vi "UI Andor.vi"(8 "error in":errorcluster) -> (0 "error out":errorcluster)   [LabVIEW 2019, in "Andor.lvlib"]
uses:
  Andor.lvlib
  User Event/Controls/UE Abort Action.ctl
  <vilib>/vision/Image Controls.llb/IMAQ Image.ctl
  <vilib>/Utility/miscctls.llb/LVPointTypeDef.ctl
  <vilib>/Utility/error.llb/Error Cluster From Error Code.vi
  <vilib>/ErrorRing/Error Ring.xnode
  Queues/Queues.lvlib
panel:
  in  "Overlay":bool
  in  "Exposure Time(s)":dbl=0.05 min=0.01 max=5.0
  out "Image":T1(plugin-control)
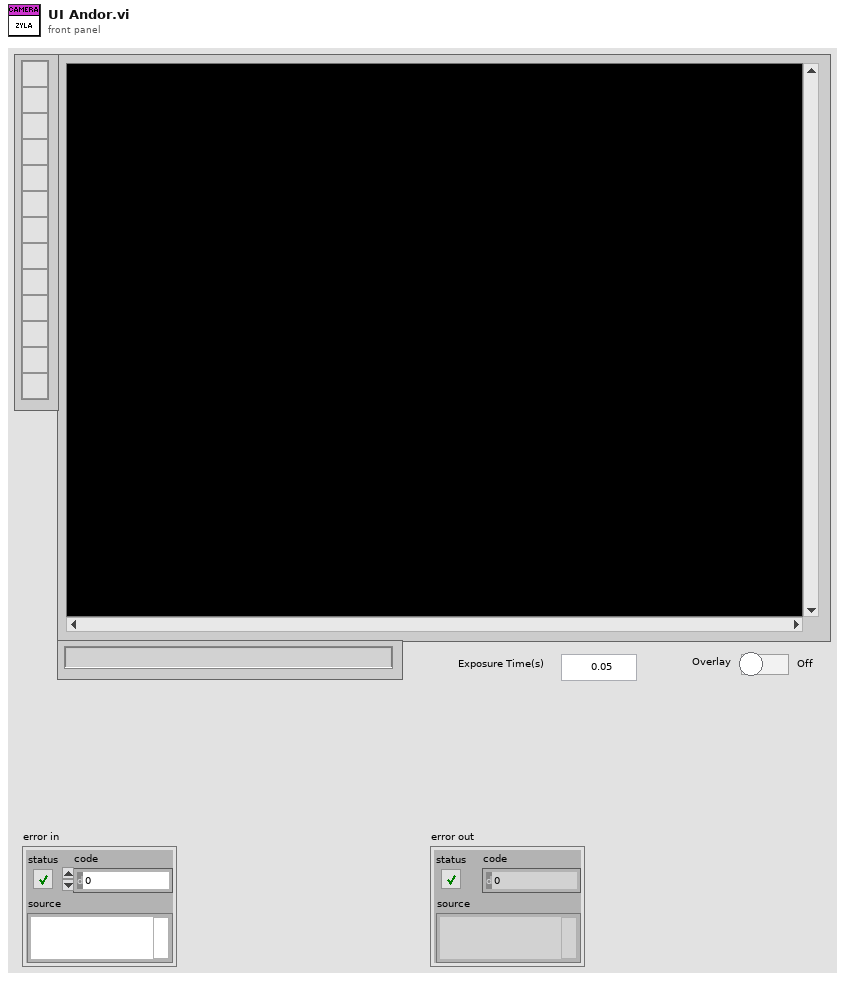
[diagram p1: front panel]
types:
  T1 = typedef "IMAQ Image.ctl" = refnum<image>
  T2 = typedef "IMAQ Point" = cluster{"X":sgl, "Y":sgl}
  T3 = cluster{"Image(U16)":T1, "Initialize Sucess?":bool, "Cursor Points":T2[], "Overlay?":bool}
  T4 = typedef "UE Abort Action.ctl" = enum16{"Create", "Get", "Destroy"}
  T5 = typedef "LVPointTypeDef.ctl" = cluster{"Horizontal":i16, "Vertical":i16}
  T6 = enum16{"Initial", "Start", "Astop", "Snap", "Exposure", "Close"}
  T7 = typedef "Image Type" = u32
  T8 = typedef "Andor.lvlib/SEQ Data.ctl" = cluster{"Initialize Sucess?":bool, "Image Ref":T1, "VI Refnum":refnum<vi>}
  T9 = typedef "Rendezvous RefNum" = refnum<k1>
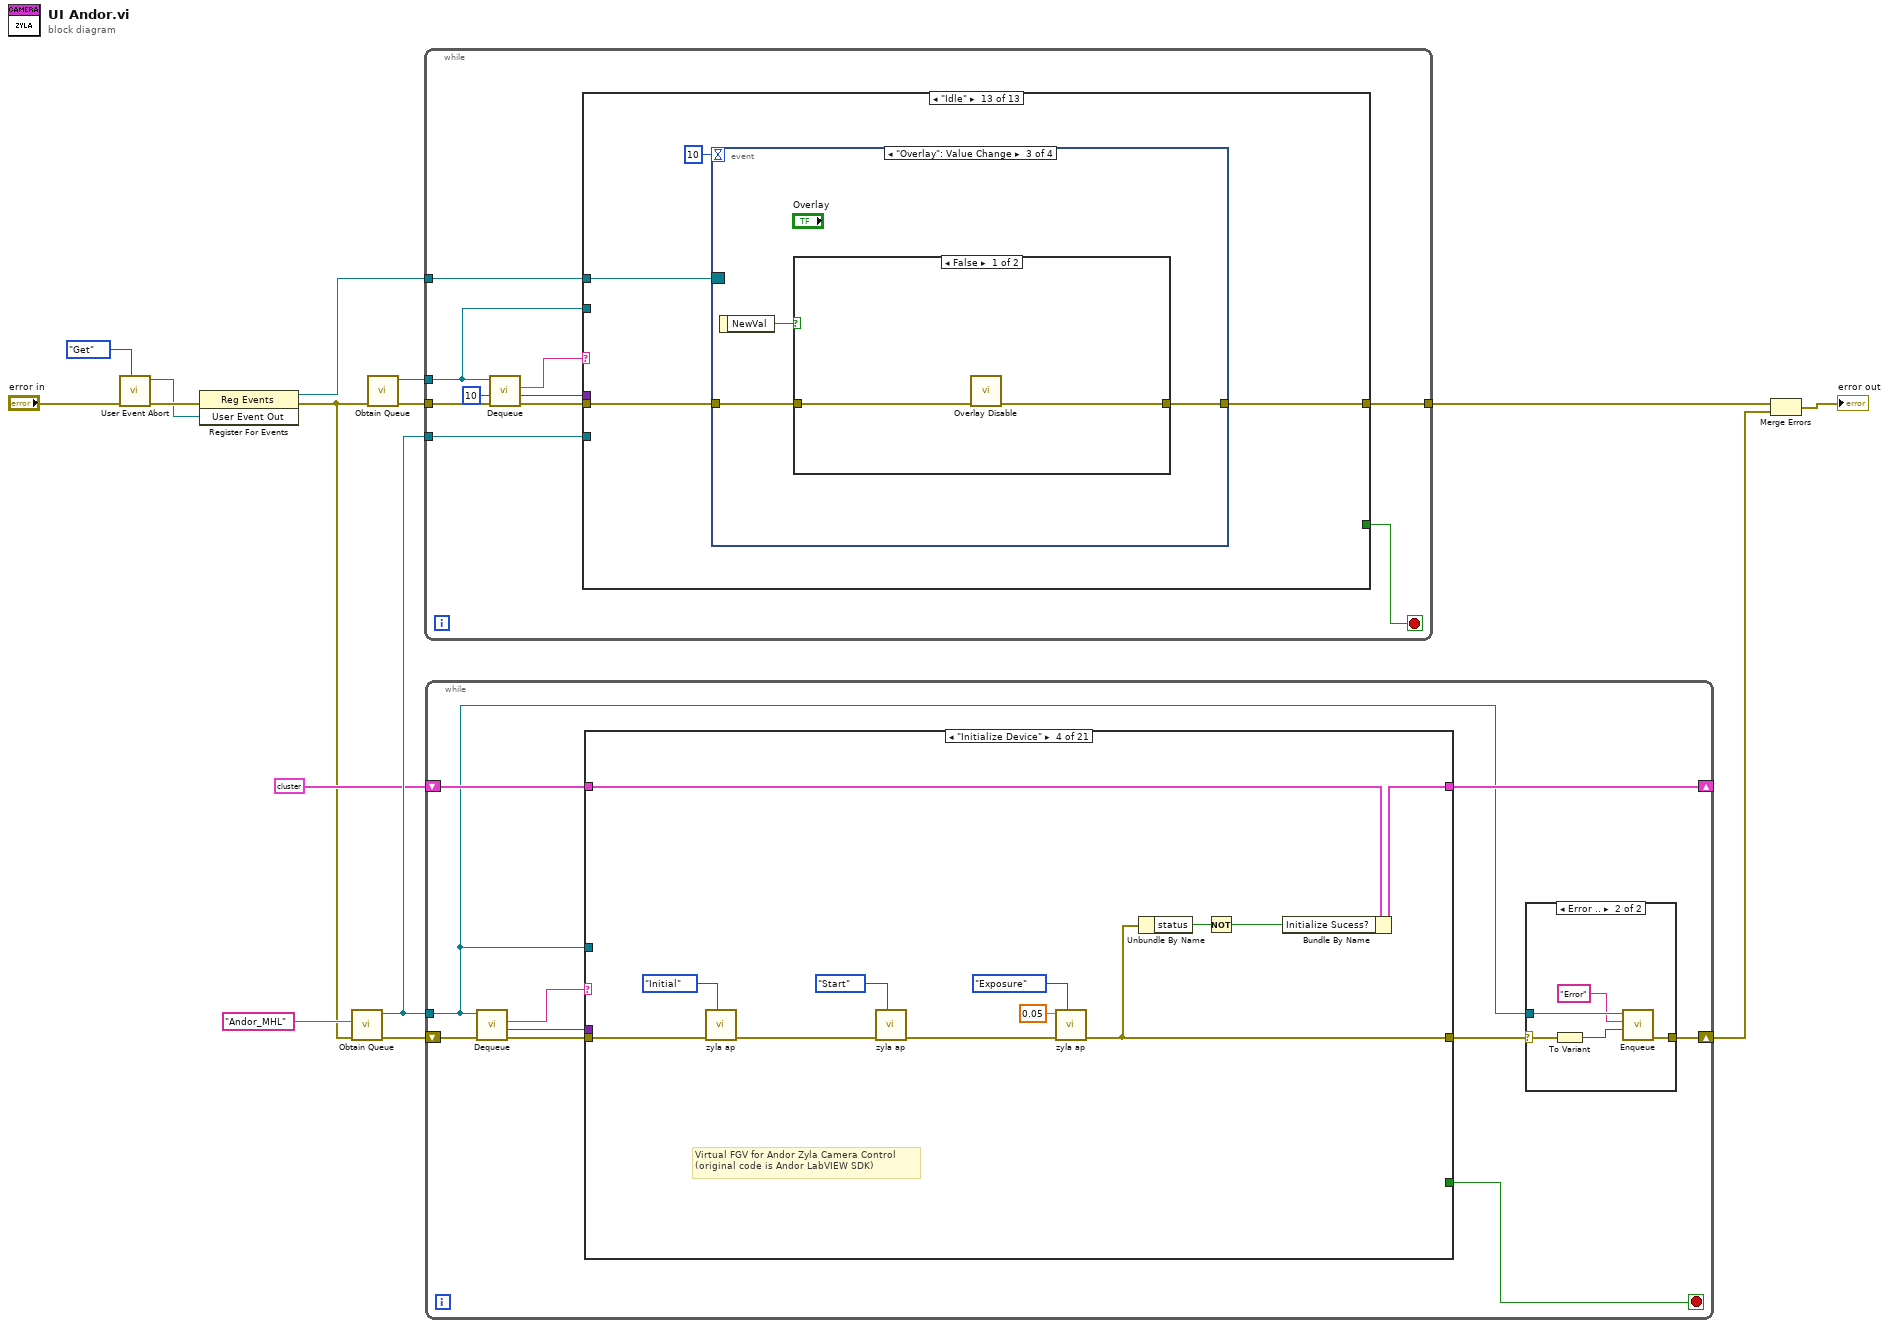
[diagram p0: block diagram]
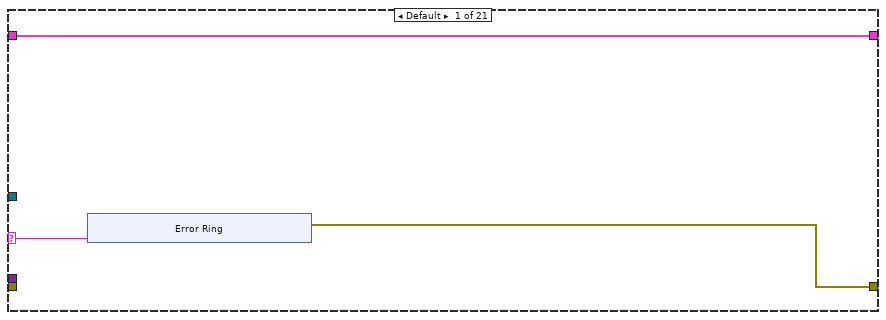
[diagram p2: hidden frame]
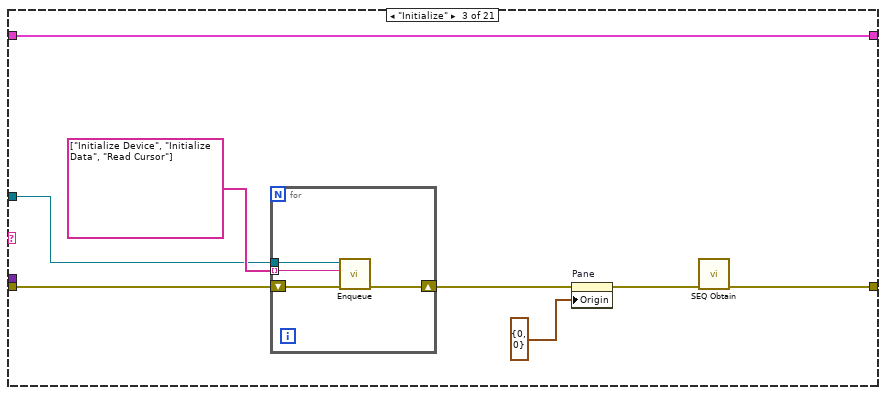
[diagram p4: hidden frame]
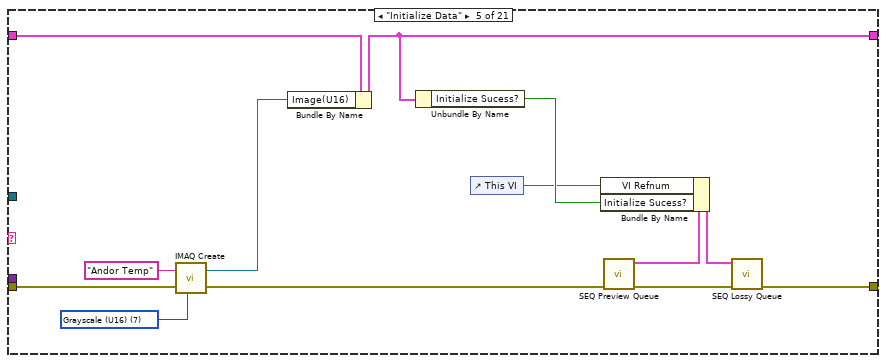
[diagram p5: hidden frame]
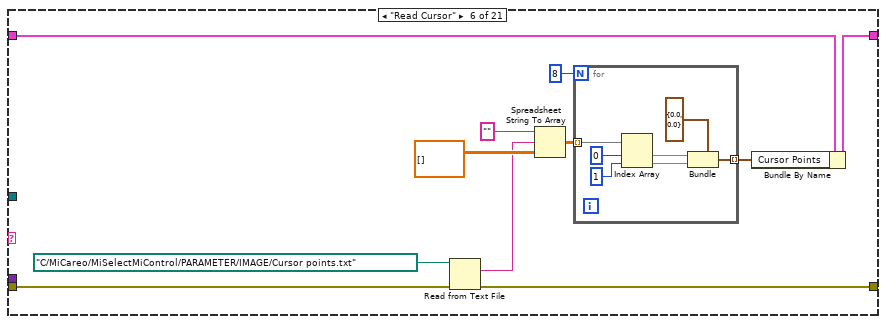
[diagram p6: hidden frame]
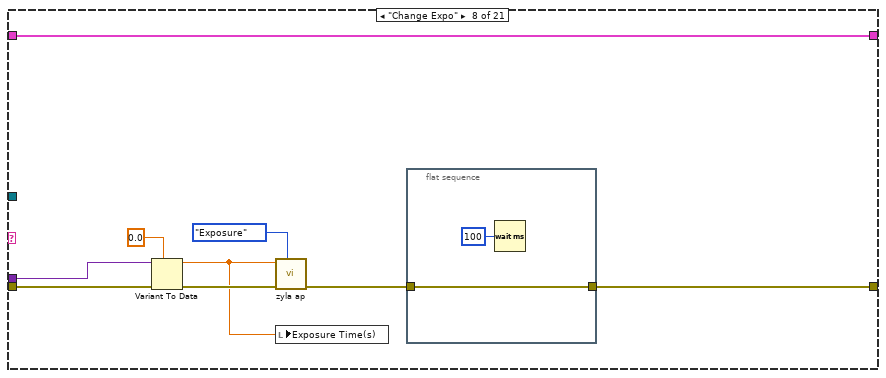
[diagram p8: hidden frame]
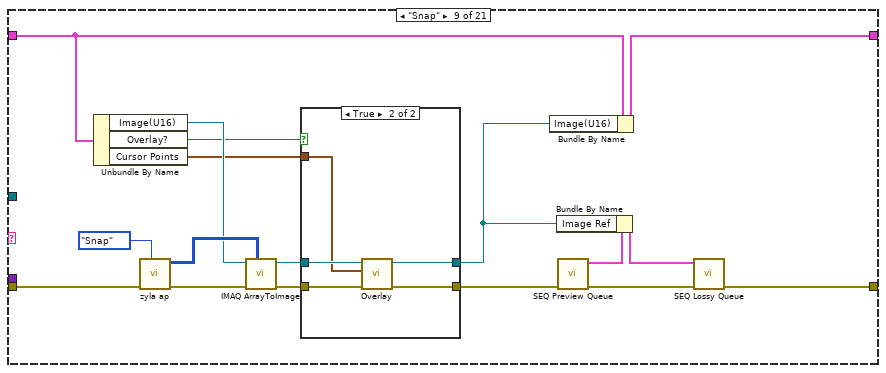
[diagram p9: hidden frame]
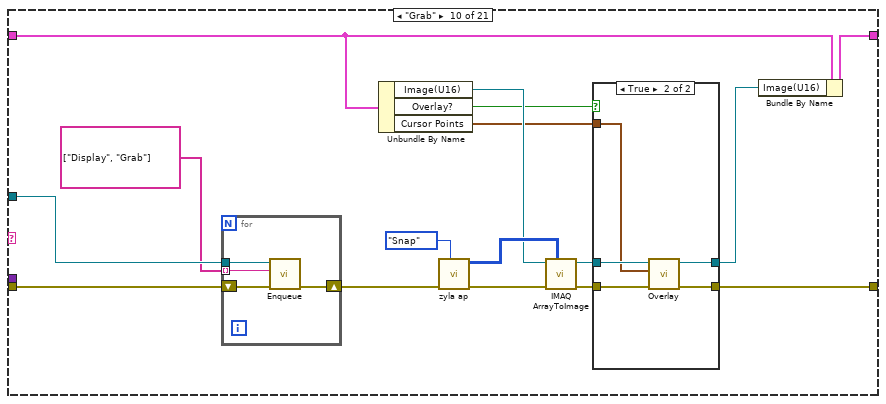
[diagram p11: hidden frame]
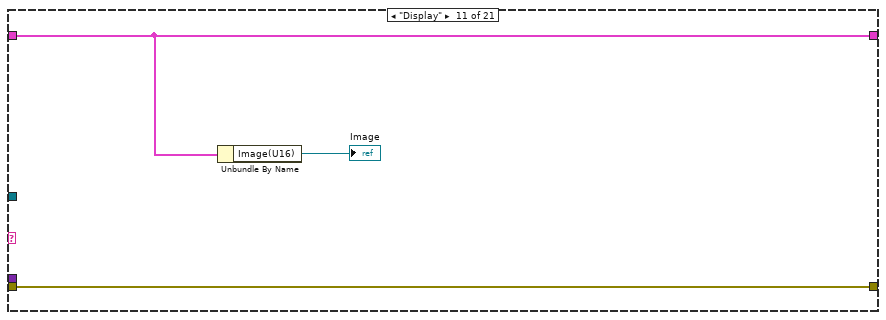
[diagram p13: hidden frame]
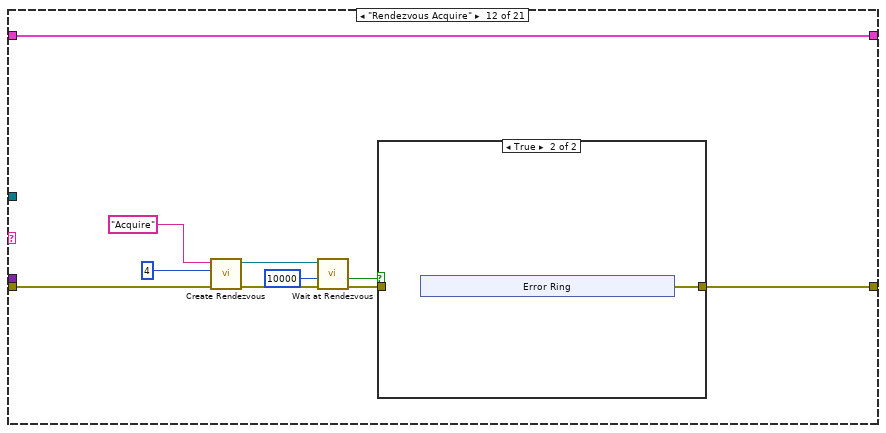
[diagram p14: hidden frame]
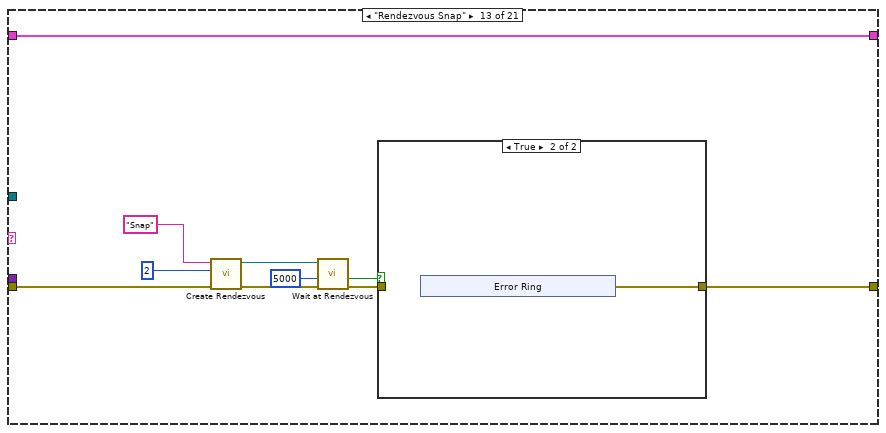
[diagram p16: hidden frame]
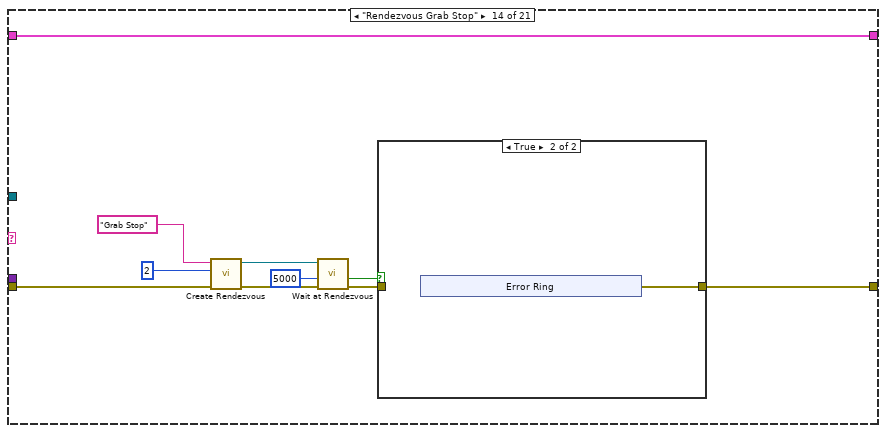
[diagram p18: hidden frame]
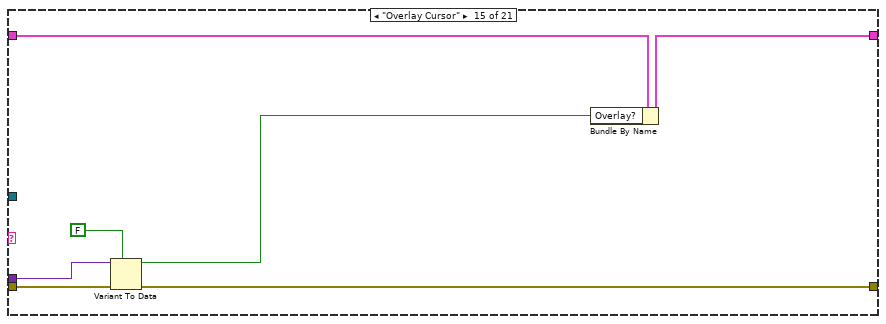
[diagram p20: hidden frame]
diagram:
  n1 = call "User Event Abort.vi"("Action"=UE_Abort_Action."Get", "Error In"="error in") -> ("Error Out"=w13:errorcluster, "User Event Out"=w12:refnum<user-event>)  [unwired: 8 in]
  n2 = register-events(error in=w13, w12) -> (reference out=w11:refnum<event-registration>, error out=w3:errorcluster)  [unwired: 1 in]
  n3 = call "Obtain Queue.vi"("Error In"=w3, "Queue Name"="Andor_MHL") -> ("Error Out"=w9:errorcluster, "queue out"=w5:refnum<queue>)  [unwired: 8 in]
  n4 = call "Obtain Queue.vi"("Error In"=w3) -> ("Error Out"=w2:errorcluster, "Queue out"=w1:refnum<queue>)  [unwired: 9 in]
  n5 = while {
    tunnel: w2 -> [w25]
    tunnel: w1 -> [w20]
    tunnel: [w19] -> w8
    tunnel: w11 -> [w18]
    tunnel: w5 -> [w16]
    stop <- w17 stop-if-true
    n6 = call "Dequeue.vi"("Error In"=w25, "timeout in ms (-1)"=10, "Queue in"=w20) -> ("Error Out"=w24:errorcluster, "Data"=w22:variant, "State"=w23:string)  [unwired: 5 in, 1 out]
    n7 = case shown="\"Idle\"" w23 {
      selector: w23 -> [w26 _ _ _ _ _ _ _ _ _ _ _ _]
      tunnel: w24 -> [w29 w33 w46 w50 w58 w61 w67 w73 w77 w81 w85 w89 w97]
      tunnel: w22 -> [_ _ w45 _ _ _ _ _ _ _ _ _ _]
      tunnel: w20 -> [_ _ _ _ _ _ _ _ _ _ _ _ _]
      tunnel: [w29 w32 w40 w49 w57 w60 w66 w72 w76 w80 w84 w88 w96] -> w19
      tunnel: w18 -> [_ _ _ _ _ _ _ _ _ _ _ _ w95]
      tunnel: [_ _ _ _ _ _ _ _ _ _ _ TRUE _] -> w17
      tunnel: w16 -> [_ w31 w42 w48 w56 w59 w65 w71 w75 w79 w83 w87 _]
      frame "Typo", Default {
        n8 = Concatenate Strings("Typo: " ("string"), w26) -> (w28:string)
        n9 = One Button Dialog(message=w28) -> ()  [unwired: 1 in, 1 out]
      }
      frame "Initialize" {
        n10 = for {
          tunnel: w31 -> [w35]
          shift-right: [w36] -> w32
          shift-left: w33 -> [w37]
          tunnel: string[] ["Initialize"] -> [w34] mode=indexing
          n11 = call "Enqueue.vi"("Error In"=w37, "State"=w34, "Queue in"=w35) -> ("Error Out"=w36:errorcluster)  [unwired: 7 in, 1 out]
        }
      }
      frame "Change Expo" {
        n12 = Variant To Data(error in=w46, type=0.0, Variant=w45) -> (data=w38:dbl, error out=w44:errorcluster)
        n13 = To Variant(anything=w38) -> (Variant=w43:variant)
        n14 = call "Enqueue.vi"("Error In"=w44, "Data"=w43, "State"="Change Expo", "Queue in"=w42) -> ("Error Out"=w40:errorcluster)  [unwired: 6 in, 1 out]
      }
      frame "Snap" {
        n15 = for {
          tunnel: w48 -> [w52]
          shift-right: [w53] -> w49
          shift-left: w50 -> [w54]
          tunnel: string[] ["Snap", "Display"] -> [w51] mode=indexing
          n16 = call "Enqueue.vi"("Error In"=w54, "State"=w51, "Queue in"=w52) -> ("Error Out"=w53:errorcluster)  [unwired: 7 in, 1 out]
        }
      }
      frame "Grab" {
        n17 = call "Enqueue.vi"("Error In"=w58, "State"="Grab", "Queue in"=w56) -> ("Error Out"=w57:errorcluster)  [unwired: 7 in, 1 out]
      }
      frame "Grab Stop" {
        n18 = Flush Queue(queue=w59, error in (no error)=w61) -> (error out=w60:errorcluster)  [unwired: 2 out]
      }
      frame "Overlay Enable" {
        n19 = To Variant(anything=TRUE) -> (Variant=w64:variant)
        n20 = call "Enqueue.vi"("Error In"=w67, "Data"=w64, "State"="Overlay Cursor", "Queue in"=w65) -> ("Error Out"=w66:errorcluster)  [unwired: 6 in, 1 out]
      }
      frame "Overlay Disable" {
        n21 = To Variant(anything=FALSE) -> (Variant=w70:variant)
        n22 = call "Enqueue.vi"("Error In"=w73, "Data"=w70, "State"="Overlay Cursor", "Queue in"=w71) -> ("Error Out"=w72:errorcluster)  [unwired: 6 in, 1 out]
      }
      frame "Rendezvous Acquire" {
        n23 = call "Enqueue.vi"("Error In"=w77, "State"="Rendezvous Acquire", "Queue in"=w75) -> ("Error Out"=w76:errorcluster)  [unwired: 7 in, 1 out]
      }
      frame "Rendezvous Snap" {
        n24 = call "Enqueue.vi"("Error In"=w81, "State"="Rendezvous Snap", "Queue in"=w79) -> ("Error Out"=w80:errorcluster)  [unwired: 7 in, 1 out]
      }
      frame "Rendezvous Grab Stop" {
        n25 = call "Enqueue.vi"("Error In"=w85, "State"="Rendezvous Grab Stop", "Queue in"=w83) -> ("Error Out"=w84:errorcluster)  [unwired: 7 in, 1 out]
      }
      frame "Close" {
        n26 = for {
          tunnel: w87 -> [w92]
          shift-right: [w93] -> w88
          shift-left: w89 -> [w94]
          tunnel: string[] ["Close"] -> [w91] mode=indexing
          n27 = call "Enqueue.vi"("Error In"=w94, "State"=w91, "Queue in"=w92) -> ("Error Out"=w93:errorcluster)  [unwired: 7 in, 1 out]
        }
      }
      frame "Idle" {
        n28 = event shown="[2] \"Overlay\": Value Change" {
          selector: w95 -> [_ _ _ w113]
          dyn-events: _ -> [_ _ _ _]
          timeout: 10 -> [_ _ _ _]
          tunnel: w97 -> [w99 w102 w104 w111]
          tunnel: [w99 w101 w103 w112] -> w96
          event Timeout {
            n29 = event-data() -> ()  [unwired: 1 in, 3 out]
          }
          event "Exposure Time(s)": Value Change {
            n30 = event-data() -> ()  [unwired: 1 in, 1 out]
            n31 = call "Change Expo.vi"("Error In"=w102, "Expo(s)"="Exposure Time(s)") -> ("Error Out"=w101:errorcluster)  [unwired: 9 in]
          }
          event "Overlay": Value Change {
            n32 = event-data() -> ("NewVal"=w105:bool)  [unwired: 1 in]
            n33 = case shown="False" w105 {
              tunnel: w104 -> [w107 w109]
              tunnel: [w106 w108] -> w103
              frame False {
                n34 = call "Overlay Disable.vi"("Error In"=w107) -> ("Error Out"=w106:errorcluster)  [unwired: 10 in]
              }
              frame True {
                n35 = call "Overlay Enable.vi"("Error In"=w109) -> ("Error Out"=w108:errorcluster)  [unwired: 10 in]
              }
            }
          }
          event User Event {
            n36 = event-data() -> ()  [unwired: 1 in, 4 out]
            n37 = call "Close.vi"("Error In"=w111) -> ("Error Out"=w110:errorcluster)  [unwired: 10 in]
            n38 = Unregister For Events(event registration refnum=w113, error in=w110) -> (error out=w112:errorcluster)
          }
        }
      }
    }
  }
  n39 = while {
    tunnel: w5 -> [w115]
    shift-right: [w118] -> _
    shift-left: T3 {"Image(U16)"=refnum, "Initialize Sucess?"=FALSE, "Cursor Points"=[], "Overlay?"=FALSE} -> [w119]
    shift-right: [w117] -> w6
    shift-left: w9 -> [w123]
    stop <- w114 stop-if-true
    n40 = call "Dequeue.vi"("Error In"=w123, "Queue in"=w115) -> ("Error Out"=w120:errorcluster, "Data"=w121:variant, "State"=w122:string)  [unwired: 6 in, 1 out]
    n41 = case shown="\"Initialize Device\"" w122 {
      selector: w122 -> [w125 _ _ _ _ _ _ _ _ _ _ _ _ _ _ _ _ _ _ _ _]
      tunnel: w115 -> [_ _ w141 _ _ _ _ _ _ w235 _ _ _ _ _ _ _ _ w328 _ w346]
      tunnel: w121 -> [_ _ _ _ _ _ _ w198 _ _ _ _ _ _ w312 _ w320 _ _ _ _]
      tunnel: w120 -> [_ w134 w142 w158 w171 w182 w192 w200 w220 w237 w257 w266 w283 w300 w314 w317 w321 w325 w329 w342 w347]
      tunnel: w119 -> [w126 w135 w140 w159 w172 w183 w191 w201 w216 w240 w256 w267 w284 w301 w315 w316 w318 w324 w326 w336 w345]
      tunnel: [w126 w135 w140 w151 w167 w174 w191 w201 w214 w238 w256 w267 w284 w301 w310 w316 w318 w324 w326 w336 w345] -> w118
      tunnel: [w124 w134 w136 w148 w164 w175 w192 w195 w212 w232 w257 w258 w275 w292 w313 w317 errorcluster {"status"=FALSE, "code"=0, "source"=""} ("Error Out") w325 w327 w337 w343] -> w116
      tunnel: [_ _ _ _ _ _ _ _ _ _ _ _ _ _ _ _ _ _ _ _ TRUE] -> w114
      frame Default {
        n42 = xnode "Error Ring"("parameter 0"=w125) -> ("error out"=w124:errorcluster)
      }
      frame "------Initialize------" {
      }
      frame "Initialize" {
        n43 = for {
          tunnel: w141 -> [w145]
          shift-right: [w146] -> w139
          shift-left: w142 -> [w147]
          tunnel: string[] ["Initialize Device", "Initialize Data", "Read Cursor"] -> [w144] mode=indexing
          n44 = call "Enqueue.vi"("Error In"=w147, "State"=w144, "Queue in"=w145) -> ("Error Out"=w146:errorcluster)  [unwired: 7 in, 1 out]
        }
        n45 = property on="Pane" class="Pane"(error in=w139, "Origin"=T5 {"Horizontal"=0, "Vertical"=0}) -> (error out=w137:errorcluster)  [unwired: 1 in, 1 out]
        n46 = call "SEQ Obtain.vi"("error in"=w137) -> ("error out"=w136:errorcluster)  [unwired: 9 in, 1 out]
      }
      frame "Initialize Device" {
        # "Virtual FGV for Andor Zyla Camera Control\n(original code is Andor LabVIEW SDK)"
        n47 = call "zyla ap.vi"("Action"=T6."Initial", "error"=w158) -> ("error out"=w157:errorcluster)  [unwired: 8 in, 1 out]
        n48 = call "zyla ap.vi"("Action"=T6."Start", "error"=w157) -> ("error out"=w154:errorcluster)  [unwired: 8 in, 1 out]
        n49 = call "zyla ap.vi"("Action"=T6."Exposure", "error"=w154, "ExposureTime"=0.05) -> ("error out"=w148:errorcluster)  [unwired: 7 in, 1 out]
        n50 = Unbundle By Name(w148) -> ("status"=w150:bool)
        n51 = Not(x=w150) -> (.not. x?=w149:bool)
        n52 = Bundle By Name(cluster=w159, "Initialize Sucess?"=w149) -> (w151:T3)
      }
      frame "Initialize Data" {
        w170 = T7 7 items=["Grayscale (U8)", "Grayscale (I16)", "Grayscale (SGL)", "Complex (CSG)", "RGB (U32)", "HSL (U32)", "RGB (U64)", "Grayscale (U16)"] ("Image Type")
        n53 = call "IMAQ Create"("Image Name"="Andor Temp", "Image Type"=w170, "error in (no error)"=w171) -> ("New Image"=w168:T1, "error out"=w166:errorcluster)  [unwired: 2 in]
        n54 = Bundle By Name(cluster=w172, "Image(U16)"=w168) -> (w167:T3)
        n55 = Unbundle By Name(w167) -> ("Initialize Sucess?"=w161:bool)
        n56 = control-ref of="This VI"() -> (w160:refnum<vi>)
        n57 = call "SEQ Preview Queue.vi"("error in"=w166) -> ("error out"=w165:errorcluster, "SEQ Data"=w163:T8)  [unwired: 9 in]
        n58 = Bundle By Name(cluster=w163, "VI Refnum"=w160, "Initialize Sucess?"=w161) -> (w162:T8)
        n59 = call "SEQ Lossy Queue.vi"("error in"=w165, "SEQ Data"=w162) -> ("error out"=w164:errorcluster)  [unwired: 9 in]
      }
      frame "Read Cursor" {
        n60 = Read from Text File(file (use dialog)=path "C:/MiCareo/MiSelectMiControl/PARAMETER/IMAGE/Cursor points.txt", error in=w182) -> (text=w176:string, error out=w175:errorcluster)  [unwired: 2 in, 2 out]
        n61 = Spreadsheet String To Array(format string="", spreadsheet string=w176, array type (2D Dbl)=sgl[][] [] ("array")) -> (array=w180:sgl[][])  [unwired: 1 in]
        n62 = for {
          N: 8 -> [_]
          tunnel: w180 -> [w189] mode=indexing
          tunnel: [w190] -> w173 mode=indexing
          n63 = Index Array(array=w189, index #1=0 ("index"), index #2=1 ("index")) -> (element #1=w188:sgl, element #2=w187:sgl)
          n64 = Bundle(cluster=T2 {"X"=0.0, "Y"=0.0} ("Point"), "X"=w188, "Y"=w187) -> (w190:T2)
        }
        n65 = Bundle By Name(cluster=w183, "Cursor Points"=w173) -> (w174:T3)
      }
      frame "------Functions------" {
      }
      frame "Change Expo" {
        n66 = Variant To Data(error in=w200, type=0.0 ("ExposureTime"), Variant=w198) -> (data=w193:dbl, error out=w199:errorcluster)
        n67 = call "zyla ap.vi"("Action"=T6."Exposure", "error"=w199, "ExposureTime"=w193) -> ("error out"=w196:errorcluster)  [unwired: 7 in, 1 out]
        n68 = local write "Exposure Time(s)"(w193) -> ()
        n69 = flat-sequence {
          tunnel: w196 -> [w203]
          tunnel: [w203] -> w195
          frame #0 {
            n70 = Wait (ms)(milliseconds to wait=u32 100) -> ()  [unwired: 1 out]
          }
        }
      }
      frame "Snap" {
        n71 = Unbundle By Name(w216) -> ("Image(U16)"=w215:T1, "Overlay?"=w209:bool, "Cursor Points"=w208:T2[])
        n72 = call "zyla ap.vi"("Action"=T6."Snap", "error"=w220) -> ("error out"=w218:errorcluster, "Intensity Graph"=w217:u16[][])  [unwired: 8 in]
        n73 = call "IMAQ ArrayToImage"("Image Pixels (U16)"=w217, "error in (no error)"=w218, "Image"=w215) -> ("error out"=w207:errorcluster, "Image Out"=w206:T1)  [unwired: 7 in]
        n74 = case shown="True" w209 {
          tunnel: w208 -> [_ w225]
          tunnel: w207 -> [w221 w227]
          tunnel: w206 -> [w222 w226]
          tunnel: [w221 w224] -> w205
          tunnel: [w222 w223] -> w204
          frame False {
          }
          frame True {
            n75 = call "Overlay.vi"("error in"=w227, "Cursor Points"=w225, "Refnum in"=w226) -> ("error out"=w224:errorcluster, "Refnum out"=w223:T1)  [unwired: 7 in]
          }
        }
        n76 = Bundle By Name(cluster=w216, "Image(U16)"=w204) -> (w214:T3)
        n77 = call "SEQ Preview Queue.vi"("error in"=w205) -> ("error out"=w213:errorcluster, "SEQ Data"=w211:T8)  [unwired: 9 in]
        n78 = Bundle By Name(cluster=w211, "Image Ref"=w204) -> (w210:T8)
        n79 = call "SEQ Lossy Queue.vi"("error in"=w213, "SEQ Data"=w210) -> ("error out"=w212:errorcluster)  [unwired: 9 in]
      }
      frame "Grab" {
        n80 = for {
          shift-right: [w253] -> w236
          shift-left: w237 -> [w254]
          tunnel: w235 -> [w252]
          tunnel: string[] ["Display", "Grab"] -> [w251] mode=indexing
          n81 = call "Enqueue.vi"("Error In"=w254, "State"=w251, "Queue in"=w252) -> ("Error Out"=w253:errorcluster)  [unwired: 7 in, 1 out]
        }
        n82 = Unbundle By Name(w240) -> ("Image(U16)"=w239:T1, "Overlay?"=w230:bool, "Cursor Points"=w229:T2[])
        n83 = call "zyla ap.vi"("Action"=T6."Snap", "error"=w236) -> ("error out"=w242:errorcluster, "Intensity Graph"=w241:u16[][])  [unwired: 8 in]
        n84 = call "IMAQ ArrayToImage"("Image Pixels (U16)"=w241, "error in (no error)"=w242, "Image"=w239) -> ("error out"=w233:errorcluster, "Image Out"=w231:T1)  [unwired: 7 in]
        n85 = case shown="True" w230 {
          tunnel: w233 -> [w244 w250]
          tunnel: [w244 w249] -> w232
          tunnel: w231 -> [w245 w248]
          tunnel: w229 -> [_ w247]
          tunnel: [w245 w246] -> w228
          frame False {
          }
          frame True {
            n86 = call "Overlay.vi"("error in"=w250, "Cursor Points"=w247, "Refnum in"=w248) -> ("error out"=w249:errorcluster, "Refnum out"=w246:T1)  [unwired: 7 in]
          }
        }
        n87 = Bundle By Name(cluster=w240, "Image(U16)"=w228) -> (w238:T3)
      }
      frame "Display" {
        n88 = Unbundle By Name(w256) -> ("Image(U16)"=→"Image":T1)
      }
      frame "Rendezvous Acquire" {
        n89 = call <vilib>:"Create Rendezvous.vi"("error in (no error)"=w266, "size (2)"=4, "name (unnamed)"="Acquire") -> ("error out"=w265:errorcluster, "rendezvous"=w262:T9)  [unwired: 2 in, 1 out]
        n90 = call <vilib>:"Wait at Rendezvous.vi"("error in (no error)"=w265, "ms timeout (-1)"=10000, "rendezvous"=w262) -> ("error out"=w260:errorcluster, "timed out"=w259:bool)  [unwired: 2 in, 1 out]
        n91 = case shown="True" w259 {
          tunnel: w260 -> [w268 _]
          tunnel: [w268 w269] -> w258
          frame False {
          }
          frame True {
            n92 = xnode "Error Ring"() -> ("error out"=w269:errorcluster)
          }
        }
      }
      frame "Rendezvous Snap" {
        n93 = call <vilib>:"Create Rendezvous.vi"("error in (no error)"=w283, "size (2)"=2, "name (unnamed)"="Snap") -> ("error out"=w282:errorcluster, "rendezvous"=w279:T9)  [unwired: 2 in, 1 out]
        n94 = call <vilib>:"Wait at Rendezvous.vi"("error in (no error)"=w282, "ms timeout (-1)"=5000, "rendezvous"=w279) -> ("error out"=w277:errorcluster, "timed out"=w276:bool)  [unwired: 2 in, 1 out]
        n95 = case shown="True" w276 {
          tunnel: w277 -> [w285 _]
          tunnel: [w285 w286] -> w275
          frame False {
          }
          frame True {
            n96 = xnode "Error Ring"() -> ("error out"=w286:errorcluster)
          }
        }
      }
      frame "Rendezvous Grab Stop" {
        n97 = call <vilib>:"Create Rendezvous.vi"("error in (no error)"=w300, "size (2)"=2, "name (unnamed)"="Grab Stop") -> ("error out"=w299:errorcluster, "rendezvous"=w296:T9)  [unwired: 2 in, 1 out]
        n98 = call <vilib>:"Wait at Rendezvous.vi"("error in (no error)"=w299, "ms timeout (-1)"=5000, "rendezvous"=w296) -> ("error out"=w294:errorcluster, "timed out"=w293:bool)  [unwired: 2 in, 1 out]
        n99 = case shown="True" w293 {
          tunnel: w294 -> [w302 _]
          tunnel: [w302 w303] -> w292
          frame False {
          }
          frame True {
            n100 = xnode "Error Ring"() -> ("error out"=w303:errorcluster)
          }
        }
      }
      frame "Overlay Cursor" {
        n101 = Variant To Data(error in=w314, type=FALSE, Variant=w312) -> (data=w309:bool, error out=w313:errorcluster)
        n102 = Bundle By Name(cluster=w315, "Overlay?"=w309) -> (w310:T3)
      }
      frame "------Error Handler------" {
      }
      frame "Error" {
        n103 = Variant To Data(error in=w321, type=errorcluster {"status"=FALSE, "code"=0, "source"=""} ("error constant"), Variant=w320) -> (data=w322:errorcluster)  [unwired: 1 out]
        n104 = call <vilib>:"Simple Error Handler.vi"("error in (no error)"=w322) -> ()  [unwired: 4 in, 5 out]
      }
      frame "------Close------" {
      }
      frame "Close" {
        n105 = for {
          tunnel: w328 -> [w332]
          shift-right: [w333] -> w327
          shift-left: w329 -> [w334]
          tunnel: string[] ["Close Device", "Release Queue"] -> [w331] mode=indexing
          n106 = call "Enqueue.vi"("Error In"=w334, "State"=w331, "Queue in"=w332) -> ("Error Out"=w333:errorcluster)  [unwired: 7 in, 1 out]
        }
      }
      frame "Close Device" {
        n107 = call "zyla ap.vi"("Action"=T6."Astop", "error"=w342) -> ("error out"=w341:errorcluster)  [unwired: 8 in, 1 out]
        n108 = Unbundle By Name(w336) -> ("Image(U16)"=w335:T1)
        n109 = call "zyla ap.vi"("Action"=T6."Close", "error"=w341) -> ("error out"=w338:errorcluster)  [unwired: 8 in, 1 out]
        n110 = call "IMAQ Dispose"("Image"=w335, "error in (no error)"=w338) -> ("error out"=w337:errorcluster)  [unwired: 4 in]
      }
      frame "Release Queue" {
        n111 = Release Queue(queue=w346, error in (no error)=w347) -> (error out=w344:errorcluster)  [unwired: 1 in, 2 out]
        n112 = call "SEQ Release Queue.vi"("error in"=w344) -> ("error out"=w343:errorcluster)  [unwired: 10 in]
      }
    }
    n113 = case shown="Error .." w116 {
      selector: w116 -> [w349 w353]
      tunnel: [w349 w354] -> w117
      tunnel: w115 -> [_ w351]
      frame No Error {
      }
      frame Error {
        n114 = To Variant(anything=w353) -> (Variant=w352:variant)
        n115 = call "Enqueue.vi"("Data"=w352, "State"="Error", "Queue in"=w351) -> ("Error Out"=w354:errorcluster)  [unwired: 7 in, 1 out]
      }
    }
  }
  n116 = Merge Errors(w8, w6) -> (→"error out":errorcluster)
